vi "test_input.vi"(7 "Config":T1={"IO params"={"Conversion"={"Rate"=4.0, "Num cards"=2, "Out channels"=4}, "Carriers"={"Phase shift"=180.0, "Levels"=[[0.8, 0.8, 0.8], [0.03, 0.03, 0.03]], "Delay samples"=73.15}, "TCP"={"Host"="192.168.1.15", "Port"=6666, "Buffering"=6, "Timeout"=6}, "Input channel sign"=[1, 1, 1]}, "High rate STFT"={"Win param"=101.5, "Window type"=61, "Win order"=2, "DFT size"=64, "Channels"=[7], "Oversample"=64}, "Low rate STFT"={"Win param"=120.0, "Window type"=61, "Win order"=8, "DFT size"=64, "Channels"=[7], "Oversample"=64}, "Filtering "=[]} {"Filtering"."Distortion"."Limit" format="%#_3p"; "Filtering"."Distortion"."LF cut" format="%#_3p"; "Filtering"."Kalman"."Measure noise" format="%#_3p"; "Filtering"."Kalman"."Process noise" format="%#_3p"; "Filtering"."Hum"."Limit" format="%#_3p"; "Filtering"."Hum"."Frequency" format="%#_4p"; "Low rate STFT"."Oversample" min=1 step=1; "Low rate STFT"."Channels" min=0 step=1; "Low rate STFT"."DFT size" min=1 step=1; "Low rate STFT"."Window type" items=["Rectangle"=0, "Hanning"=1, "Hamming"=2, "Blackman-Harris"=3, "Exact Blackman"=4, "Blackman"=5, "Flat Top"=6, "4 Term B-Harris "=7, "7 Term B-Harris"=8, "Low Sidelobe"=9, "Blackman Nuttall"=11, "Triangle"=30, "Bartlett-Hanning"=31, "Bohman"=32, "Parzen"=33, "Welch"=34, "Kaiser"=60, "Dolph-Chebyshev"=61, "Gaussian"=62]; "High rate STFT"."Oversample" min=1 step=1; "High rate STFT"."Channels" min=0 step=1; "High rate STFT"."DFT size" min=1 step=1; "High rate STFT"."Window type" items=["Rectangle"=0, "Hanning"=1, "Hamming"=2, "Blackman-Harris"=3, "Exact Blackman"=4, "Blackman"=5, "Flat Top"=6, "4 Term B-Harris "=7, "7 Term B-Harris"=8, "Low Sidelobe"=9, "Blackman Nuttall"=11, "Triangle"=30, "Bartlett-Hanning"=31, "Bohman"=32, "Parzen"=33, "Welch"=34, "Kaiser"=60, "Dolph-Chebyshev"=61, "Gaussian"=62]; "IO params"."Input channel sign" min=-1 max=1 step=1; "IO params"."Carriers"."Levels" min=0.0 step=0.1; "IO params"."Conversion"."Rate" format="%#_8g"}, 11 "data in":waveform(dbl)[][](array[waveform])) -> (0 "Clipping":bool, 1 "I RMS":dbl[](array[numeric]) format="%.3g", 3 "Raw data":dbl[][][](array[numeric]), 4 "Drive low":bool)   [LabVIEW 2026]
uses:
  processing/ilemt_config.ctl
  system/IO_params.ctl
  processing/stft_params.ctl
  <vilib>/Analysis/4window.llb/windowTd.ctl
  processing/filter_params.ctl
  processing/detrend_mode.ctl
  <vilib>/Analysis/NI_AALPro.lvlib
panel:
  in  "Saved Full scale current (A)  for hi power out":dbl[](array[numeric])=[16.34, 16.34, 16.34]
  in  "Low drive threshold":dbl=0.05
  in  "Full scale current (A)":dbl[](array[numeric])=[0.488, 0.488, 0.488]
  # "Page is the card number, where current sense is card 0, and later cards are for sensors.  The row is XYZ and the column is sample."
  # "Convert data from waveform array to 3D array and extract amps current, clipping."
  # "Parameter:"
  # "(was 2.0 for high power out)"
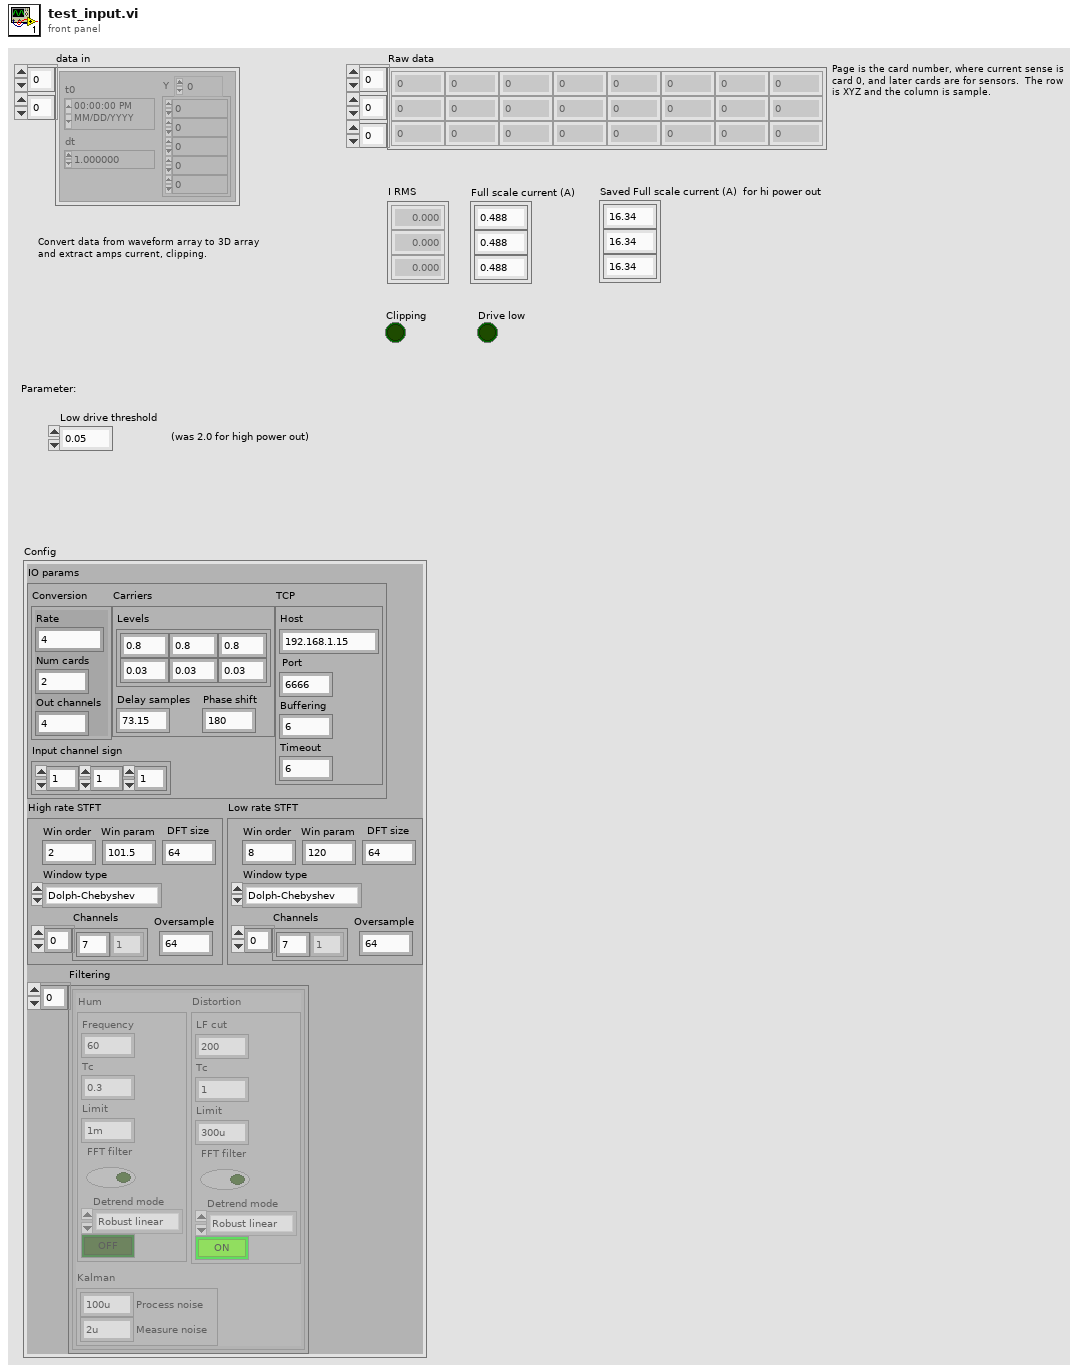
[diagram p1: front panel]
types:
  T1 = typedef "ilemt_config.ctl" = cluster{"IO params":T2, "High rate STFT":T3, "Low rate STFT":T3, "Filtering ":T5[]}
  T2 = typedef "IO_params.ctl" = cluster{"Conversion":cluster{"Rate":dbl, "Num cards":u32, "Out channels":u32}, "Carriers":cluster{"Phase shift":dbl, "Levels":dbl[][], "Delay samples":dbl}, "TCP":cluster{"Host":string, "Port":i32, "Buffering":u32, "Timeout":u32}, "Input channel sign":i32[]}
  T3 = typedef "stft_params.ctl" = cluster{"Win param":dbl, "Window type":T4, "Win order":i32, "DFT size":i32, "Channels":i32[], "Oversample":i32}
  T4 = typedef "NI_AALPro.lvlib/windowTd.ctl" = u32
  T5 = typedef "filter_params.ctl" = cluster{"Hum":cluster{"Frequency":dbl, "Tc":dbl, "Limit":dbl, "FFT filter":bool, "Detrend mode":T6, "Enable":bool}, "Kalman":cluster{"Process noise":dbl, "Measure noise":dbl}, "Distortion":cluster{"LF cut":dbl, "Tc":dbl, "Limit":dbl, "FFT filter":bool, "Detrend mode":T6, "Enable":bool}}
  T6 = typedef "detrend_mode.ctl" = enum16{"Zero mean", "Linear", "Robust linear"}
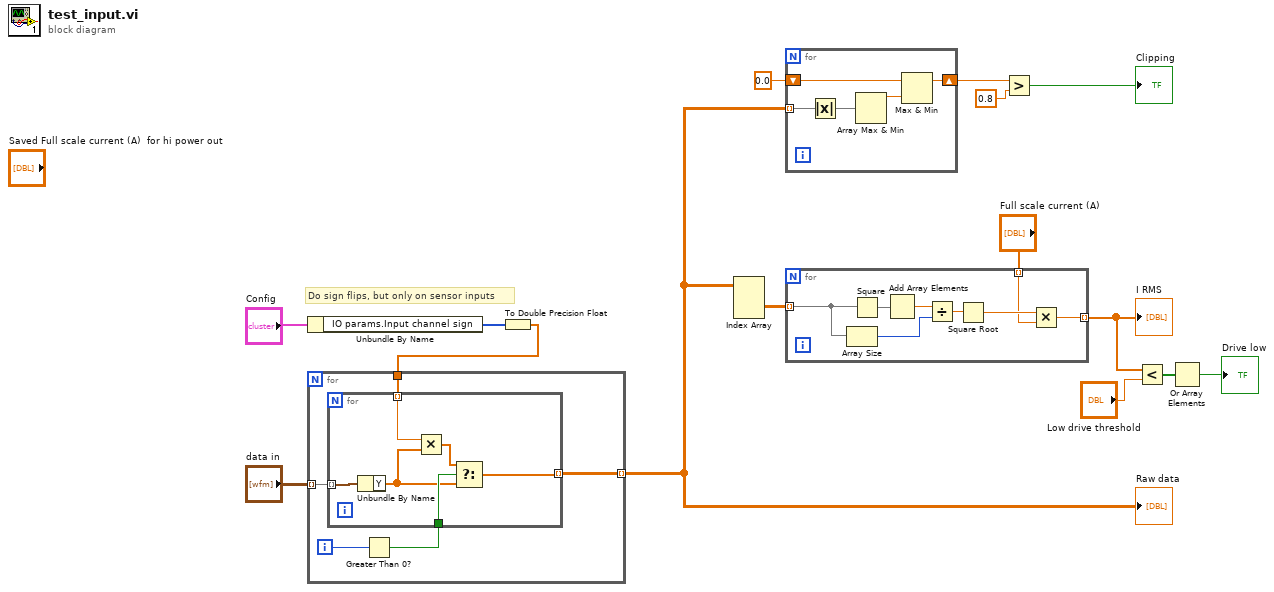
[diagram p0: block diagram]
diagram:
  # "Do sign flips, but only on sensor inputs"
  n1 = Unbundle By Name("Config") -> ("IO params.Input channel sign"=w2:i32[])
  n2 = To Double Precision Float(number=w2) -> (double precision float=w1:dbl[])
  n3 = for {
    tunnel: "data in" -> [w20] mode=indexing
    tunnel: [w19] -> w8 mode=indexing
    tunnel: w1 -> [w16]
    i -> [w18]
    n4 = Greater Than 0?(x=w18) -> (x > 0?=w17:bool)
    n5 = for {
      tunnel: w20 -> [w26] mode=indexing
      tunnel: [w24] -> w19 mode=indexing
      tunnel: w17 -> [w25]
      tunnel: w16 -> [w21] mode=indexing
      n6 = Unbundle By Name(w26) -> ("Y"=w22:dbl[])
      n7 = Multiply(x=w21, y=w22) -> (x*y=w23:dbl[])
      n8 = Select(t=w23, s=w25, f=w22) -> (s? t:f=w24:dbl[])
    }
  }
  "Raw data" <- w8
  n9 = Index Array(array=w8) -> (element=w9:dbl[][])  [unwired: 3 in]
  n10 = for {
    tunnel: w8 -> [w28] mode=indexing
    shift-right: [w29] -> w13
    shift-left: 0.0 -> [w30]
    n11 = Absolute Value(x=w28) -> (abs(x)=w27:dbl[][])
    n12 = Array Max & Min(array=w27) -> (max value=w31:dbl)  [unwired: 3 out]
    n13 = Max & Min(x=w30, y=w31) -> (max(x,y)=w29:dbl)  [unwired: 1 out]
  }
  n14 = for {
    tunnel: [w35] -> w7 mode=indexing
    tunnel: w9 -> [w32] mode=indexing
    tunnel: "Full scale current (A)" -> [w33] mode=indexing
    n15 = Array Size(array=w32) -> (size(s)=w39:i32)
    n16 = Square(x=w32) -> (x^2=w36:dbl[])
    n17 = Add Array Elements(numeric array=w36) -> (sum=w37:dbl)
    n18 = Divide(x=w37, y=w39) -> (x/y=w38:dbl)
    n19 = Square Root(x=w38) -> (sqrt(x)=w34:dbl)
    n20 = Multiply(x=w34, y=w33) -> (x*y=w35:dbl)
  }
  "I RMS" <- w7
  n21 = Greater?(x=w13, y=0.8) -> (0:→"Clipping":bool)
  n22 = Less?(x=w7, y="Low drive threshold") -> (x < y?=w5:bool[])
  n23 = Or Array Elements(Boolean array=w5) -> (logical OR=→"Drive low":bool)
